vi "MessungKlimadaten(SubVI).vi"(4 "Datei LV-Interpretation":refnum<file>, 6 "Datei COM":refnum<file>, 7 "Boolesch":bool, 8 "Fehler (Eingang, kein Fehler)":errorcluster, 9 "VISA resource name out":refnum<visa-resource-name>, 10 "Lufttemperatur [°C] (Eingang)":refnum<vi>, 11 "Luftdruck [mbar] (Eingang)":refnum<vi>) -> (0 "Fehler (Ausgang)":errorcluster, 3 "VISA-Referenz (Ausgang)":refnum<visa-resource-name>)   [LabVIEW 2014]
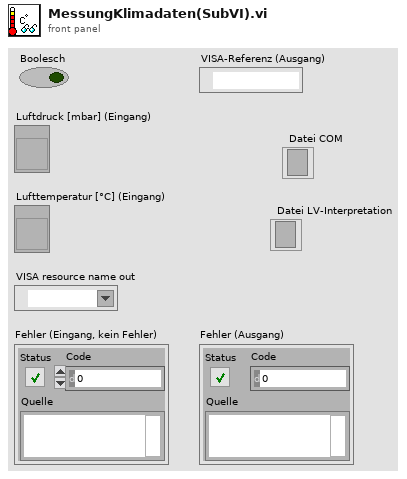
[diagram p1: front panel]
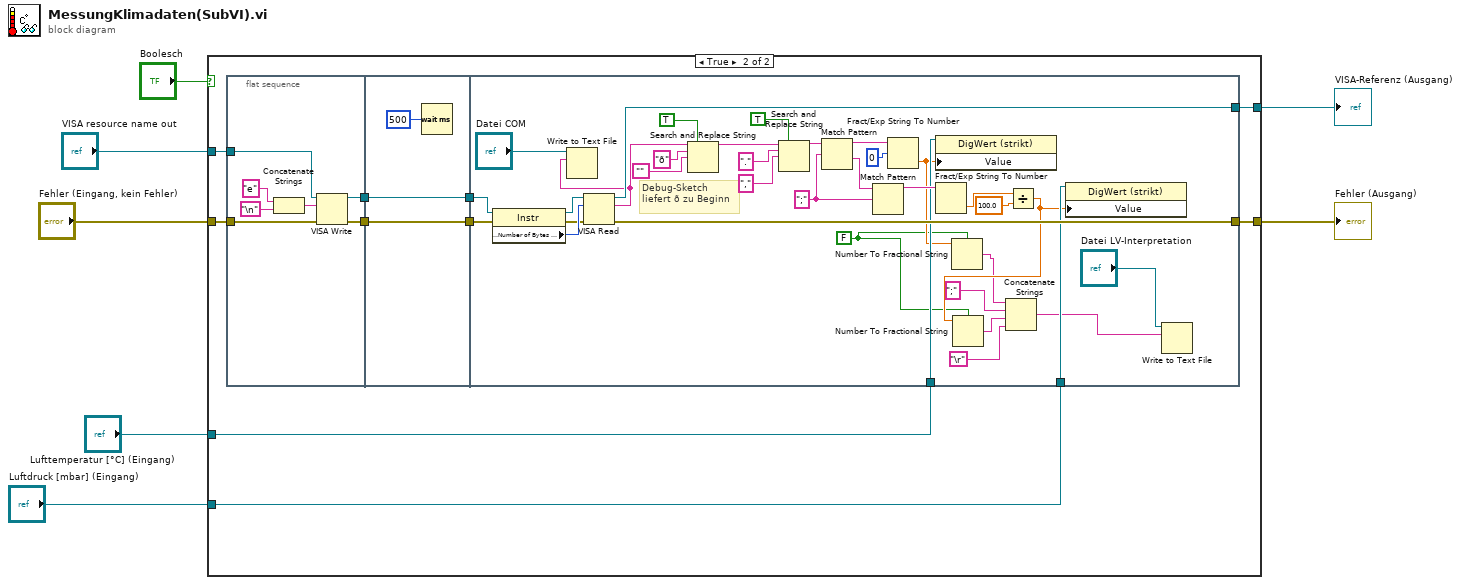
[diagram p0: block diagram]
diagram:
  n1 = case shown="True" "Boolesch" {
    tunnel: [w9 w12] -> w3
    tunnel: [w8 w13] -> w4
    tunnel: "VISA resource name out" -> [w9 w19]
    tunnel: "Fehler (Eingang, kein Fehler)" -> [w8 w18]
    tunnel: "Luftdruck [mbar] (Eingang)" -> [_ w11]
    tunnel: "Lufttemperatur [°C] (Eingang)" -> [_ w10]
    frame False {
    }
    frame True {
      n2 = flat-sequence {
        tunnel: w19 -> [w24]
        tunnel: w18 -> [w23]
        tunnel: [w26] -> w17
        tunnel: [w25] -> w16
        tunnel: w17 -> [w29]
        tunnel: w16 -> [w28]
        tunnel: [w29] -> w15
        tunnel: [w28] -> w14
        tunnel: w15 -> [w51]
        tunnel: w14 -> [w50]
        tunnel: [w53] -> w13
        tunnel: [w52] -> w12
        tunnel: w11 -> [w49]
        tunnel: w10 -> [w48]
        frame #0 {
          n3 = Concatenate Strings("e" ("String"), "\n") -> (w22:string)
          n4 = VISA Write(VISA resource name=w24, write buffer=w22, error in (no error)=w23) -> (VISA resource name out=w26:refnum<visa-resource-name>, error out=w25:errorcluster)  [unwired: 1 out]
        }
        frame #1 {
          n5 = Wait (ms)(milliseconds to wait=u32 500 ("Zu wartende ms")) -> ()  [unwired: 1 out]
        }
        frame #2 {
          w30 = FALSE
          w57 = ";" ("Regulärer Ausdruck")
          # "Debug-Sketch liefert ð zu Beginn"
          n6 = property class="Instr"(reference=w51, error in=w50) -> (reference out=w58:refnum<visa-resource-name>, error out=w59:errorcluster, "Serial Settings:Number of Bytes at Serial Port"=w60:u32)
          n7 = VISA Read(VISA resource name=w58, byte count=w60, error in (no error)=w59) -> (VISA resource name out=w52:refnum<visa-resource-name>, read buffer=w40:string, error out=w53:errorcluster)  [unwired: 1 out]
          n8 = Write to Text File(file (use dialog)="Datei COM", text=w40) -> ()  [unwired: 2 in, 3 out]
          n9 = Search and Replace String(replace all?=TRUE ("Alle ersetzen? (F)"), input string=w40, search string="ð" ("Such-String"), replace string="") -> (result string=w42:string)  [unwired: 4 in, 3 out]
          n10 = Search and Replace String(replace all?=TRUE ("Alle ersetzen? (F)"), input string=w42, search string="." ("Such-String"), replace string="," ("Ersetzungs-String (\"\")")) -> (result string=w62:string)  [unwired: 4 in, 3 out]
          n11 = Match Pattern(string=w62, regular expression=w57) -> (before substring=w45:string, after substring=w63:string)  [unwired: 1 in, 2 out]
          n12 = Match Pattern(string=w63, regular expression=w57) -> (before substring=w64:string)  [unwired: 1 in, 3 out]
          n13 = Fract/Exp String To Number(string=w45, offset=0 ("Offset")) -> (number=w32:dbl)  [unwired: 2 in, 1 out]
          n14 = property class="DigWert (strikt)"(reference=w48, "Value"=w32) -> ()  [unwired: 1 in, 2 out]
          n15 = Fract/Exp String To Number(string=w64) -> (number=w61:dbl)  [unwired: 3 in, 1 out]
          n16 = Number To Fractional String(use system decimal point (T)=w30, number=w32) -> (F-format string=w31:string)  [unwired: 2 in]
          n17 = Divide(x=w61, y=100.0 ("x")) -> (x/y=w38:dbl)
          n18 = Number To Fractional String(use system decimal point (T)=w30, number=w38) -> (F-format string=w37:string)  [unwired: 2 in]
          n19 = Concatenate Strings(w31, ";", w37, "\r") -> (w35:string)
          n20 = property class="DigWert (strikt)"(reference=w49, "Value"=w38) -> ()  [unwired: 1 in, 2 out]
          n21 = Write to Text File(file (use dialog)="Datei LV-Interpretation", text=w35) -> ()  [unwired: 2 in, 3 out]
        }
      }
    }
  }
  "Fehler (Ausgang)" <- w4
  "VISA-Referenz (Ausgang)" <- w3
